vi "Check for Mirrors.vi"(5 "Ny":i32, 7 "Nx":i32, 9 "yPrev":u64, 10 "xPrev":u64, 11 "Rocks":cluster{i32, i32}[](array[cluster])) -> (0 "Horizontal Mirror?":bool, 1 "Mirrored Rows":u64, 2 "Vertical Mirror?":bool, 3 "Mirrored Columns":u64)   [LabVIEW 2023, in "d13.lvlib"]
uses:
  d13.lvlib
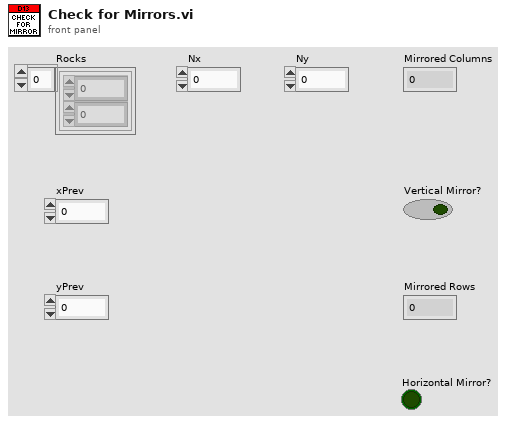
[diagram p1: front panel]
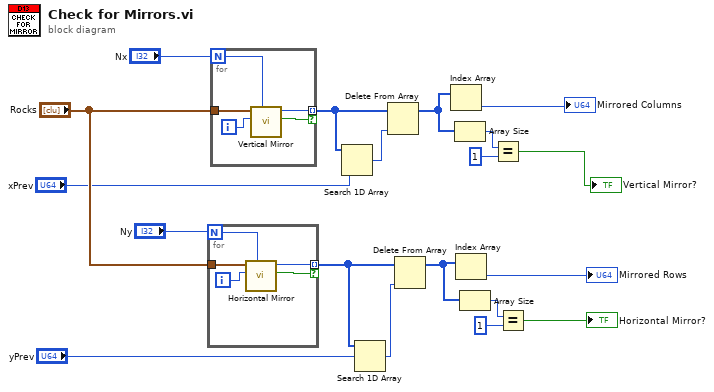
[diagram p0: block diagram]
diagram:
  n1 = for {
    N: "Ny" -> [w24]
    tunnel: "Rocks" -> [w23]
    tunnel: [w21] -> w4 mode=indexing if=w20
    i -> [w22]
    n2 = call "Horizontal Mirror.vi"("N"=w24, "Mirror Position"=w22, "Rocks"=w23) -> ("Mirror?"=w20:bool, "Rows"=w21:u64)  [unwired: 7 in]
  }
  n3 = for {
    N: "Nx" -> [w26]
    tunnel: [w29] -> w8 mode=indexing if=w25
    tunnel: "Rocks" -> [w27]
    i -> [w28]
    n4 = call "Vertical Mirror.vi"("N"=w26, "Mirror Position"=w28, "Rocks"=w27) -> ("Mirror?"=w25:bool, "Mirrored Columns"=w29:u64)  [unwired: 7 in]
  }
  n5 = Search 1D Array(1D array=w8, element="xPrev") -> (index of element=w5:i32)  [unwired: 1 in]
  n6 = Search 1D Array(1D array=w4, element="yPrev") -> (index of element=w2:i32)  [unwired: 1 in]
  n7 = Delete From Array(array=w8, index=w5) -> (array with subset deleted=w6:u64[])  [unwired: 1 in, 1 out]
  n8 = Delete From Array(array=w4, index=w2) -> (array with subset deleted=w3:u64[])  [unwired: 1 in, 1 out]
  n9 = Index Array(array=w6) -> (element=→"Mirrored Columns":u64)  [unwired: 1 in]
  n10 = Array Size(array=w6) -> (size(s)=w15:i32)
  n11 = Index Array(array=w3) -> (element=→"Mirrored Rows":u64)  [unwired: 1 in]
  n12 = Array Size(array=w3) -> (size(s)=w13:i32)
  n13 = Equal?(x=w15, y=1) -> (x = y?=→"Vertical Mirror?":bool)
  n14 = Equal?(x=w13, y=1) -> (x = y?=→"Horizontal Mirror?":bool)
